vi "CRYOpen Wave File.vi"(11 "Wave File Path In":path) -> (0 "Error Out(0-OK)":u32, 1 "Wave Data Out":sgl[](array[numeric]), 2 "dT":dbl, 3 "Fs":dbl, 4 "X0":dbl, 6 "Channels":u32)   [LabVIEW 2013]
uses:
  CRYSound.dll
panel:
  in  "TaskID":u32
  in  "Samples":u32
  in  "Channel":u32
  in  "Sampling Bit":u32
  in  "Sampling Freq":u32
  # "Open Wave File."
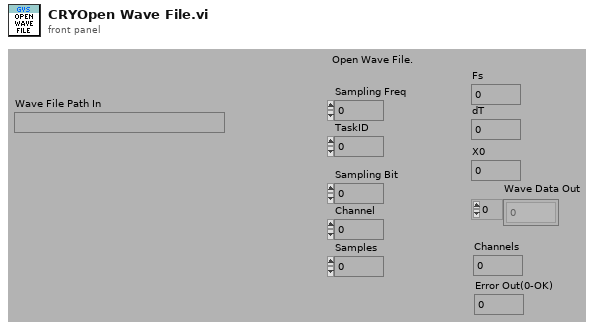
[diagram p1: front panel]
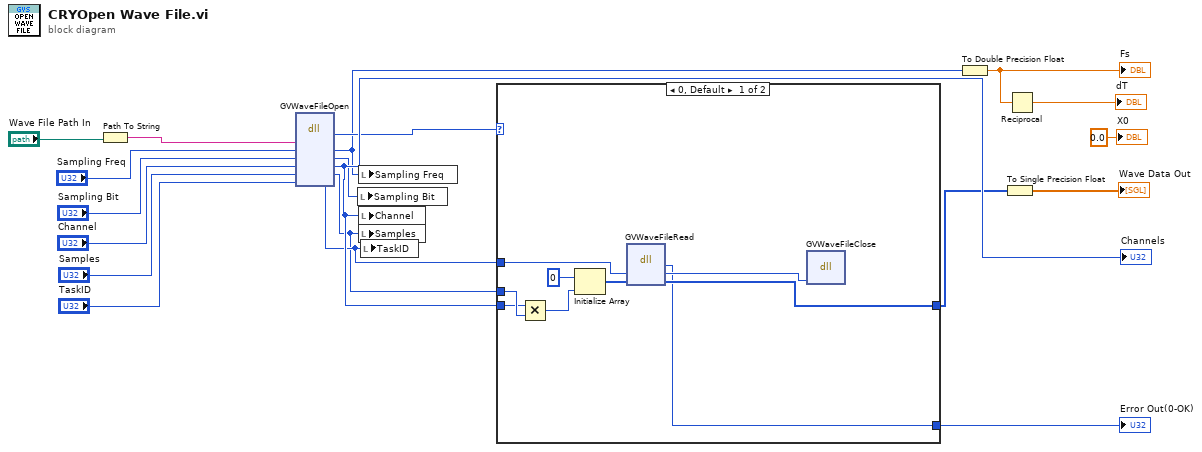
[diagram p0: block diagram]
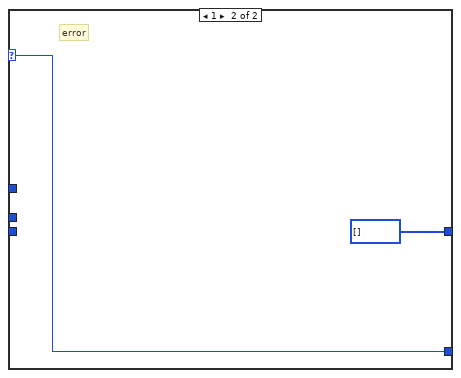
[diagram p2: hidden frame]
diagram:
  n1 = Path To String(path="Wave File Path In") -> (string=w18:string)
  n2 = dll-call lib="D:/LabView_Project/CRY6181/CRYSound.dll" fn="GVWaveFileOpen"("WaveFileName"=w18, "SampleFreq"="Sampling Freq", "BitDepth"="Sampling Bit", "nChannels"="Channel", "Samples"="Samples", "ntaskID"="TaskID") -> ("return type"=w6:u32, "SampleFreq"=w4:u32, "BitDepth"=w3:u32, "nChannels"=w7:u32, "Samples"=w1:u32, "ntaskID"=w2:u32)  [unwired: 4 in, 2 out]
  "Channels" <- w7
  n3 = local write "Sampling Bit"(w3) -> ()
  n4 = local write "Sampling Freq"(w4) -> ()
  n5 = local write "Channel"(w7) -> ()
  n6 = local write "Samples"(w1) -> ()
  n7 = local write "TaskID"(w2) -> ()
  n8 = case shown="0, Default" w6 {
    selector: w6 -> [_ w30]
    tunnel: w2 -> [w26 _]
    tunnel: [w25 i32[] [] ("pSampleData")] -> w5
    tunnel: [w23 w30] -> w17
    tunnel: w1 -> [w22 _]
    tunnel: w7 -> [w21 _]
    frame 0, Default {
      n9 = Multiply(x=w21, y=w22) -> (x*y=w20:u32)
      n10 = Initialize Array(0 ("element"), w20) -> (w27:i32[])
      n11 = dll-call lib="D:/LabView_Project/CRY6181/CRYSound.dll" fn="GVWaveFileRead"("ntaskID"=w26, "pSampleData"=w27) -> ("return type"=w23:u32, "ntaskID"=w24:u32, "pSampleData"=w25:i32[])  [unwired: 3 in, 2 out]
      n12 = dll-call lib="D:/LabView_Project/CRY6181/CRYSound.dll" fn="GVWaveFileClose"("ntaskID"=w24) -> ()  [unwired: 4 in, 3 out]
    }
    frame 1 {
      # "error"
    }
  }
  "Error Out(0-OK)" <- w17
  n13 = To Double Precision Float(number=w4) -> (double precision float=w8:dbl)
  "Fs" <- w8
  n14 = To Single Precision Float(number=w5) -> (single precision float=→"Wave Data Out":sgl[])
  n15 = Reciprocal(x=w8) -> (1/x=→"dT":dbl)
  "X0" <- 0.0 ("X0")
